vi "Framework_Initialize.vi"(8 "error in (no error)":errorcluster, 11 "AB_DepDLL in":refnum<class "AB_DepDLL.lvclass">) -> (0 "error out":errorcluster, 1 "helpTopics":string[](array[string]), 2 "pageTitles":string[](array[string]), 3 "AB_DepDLL out":refnum<class "AB_DepDLL.lvclass">, 4 "helpFile":string, 5 "pages":path[](array[path]))   [LabVIEW 2020, in "AB_DepDLL.lvclass"]
uses:
  <vilib>/AppBuilder/AB_Classes/DepDLL/AB_DepDLL.lvclass
  <vilib>/AppBuilder/AB_Classes/DLL/AB_DLL.lvclass
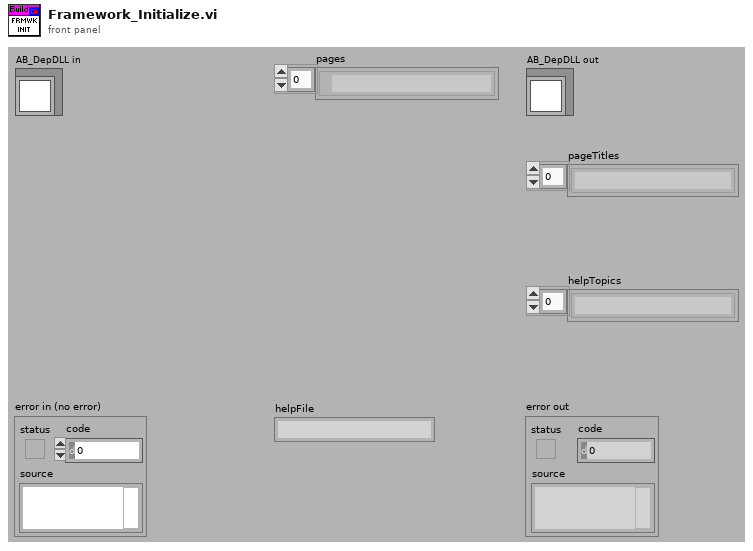
[diagram p1: front panel]
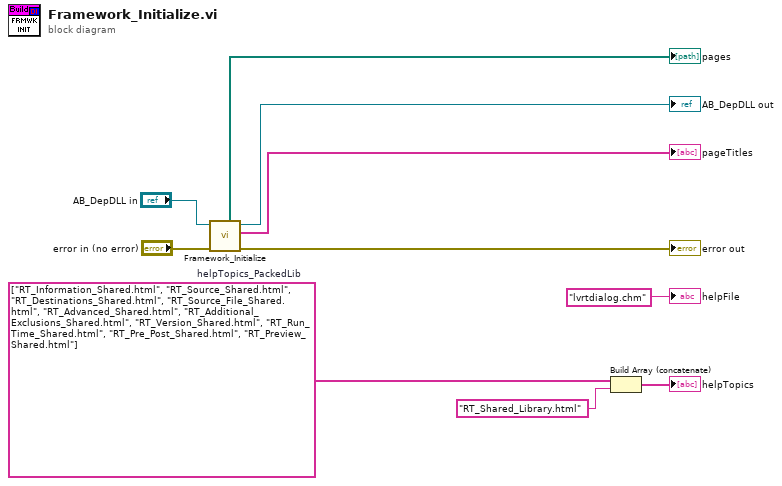
[diagram p0: block diagram]
diagram:
  w3 = string[] ["RT_Information_Shared.html", "RT_Source_Shared.html", "RT_Destinations_Shared.html", "RT_Source_File_Shared.html", "RT_Advanced_Shared.html", "RT_Additional_Exclusions_Shared.html", "RT_Version_Shared.html", "RT_Run_Time_Shared.html", "RT_Pre_Post_Shared.html", "RT_Preview_Shared.html"]  # helpTopics_PackedLib
  n1 = call-parent "Framework_Initialize.vi"("error in (no error)"="error in (no error)", "AB_DLL in"="AB_DepDLL in") -> ("error out"=→"error out":errorcluster, "pageTitles"=→"pageTitles":string[], "AB_DLL out"=→"AB_DepDLL out":refnum<class "AB_DepDLL.lvclass">, "pages"=→"pages":path[])  [unwired: 4 in, 2 out]
  n2 = Build Array (concatenate)(w3, "RT_Shared_Library.html" ("HTML filename")) -> (→"helpTopics":string[])
  "helpFile" <- "lvrtdialog.chm" ("CHM or HLP filename (lvdialog.chm)")
